vi "数据查询_数据查询.vi"() -> ()   [LabVIEW 2016]
uses:
  <vilib>/Utility/miscctls.llb/LVPointTypeDef.ctl
  <vilib>/Utility/miscctls.llb/LVRowAndColumnUnsignedTypeDef.ctl
  <userlib>/_OpenG.lib/array/array.llb/Sort 2D Array (String)__ogtk.vi
  <vilib>/addons/database/_DB Variant To Data/Database Variant To Data.xnode
panel:
  in  "导出":bool
  out "分钟小时":string(combo)="实时数据"
  out "工作类型":string(combo)="全部数据"
  in  "工作模式":string(combo)="全部数据"
  out "连接的字符串":string
  out "选中数据表":string
  in  "查询":bool
  in  "结束日期":string="2020/01/01"
  in  "起始日期":string="2010/01/01"
  out "XY图":cluster{"data":timestamp[], "data":dbl[]}[](graph)
  in  "组合框":string(combo)
  out "数据表":string[][](table)
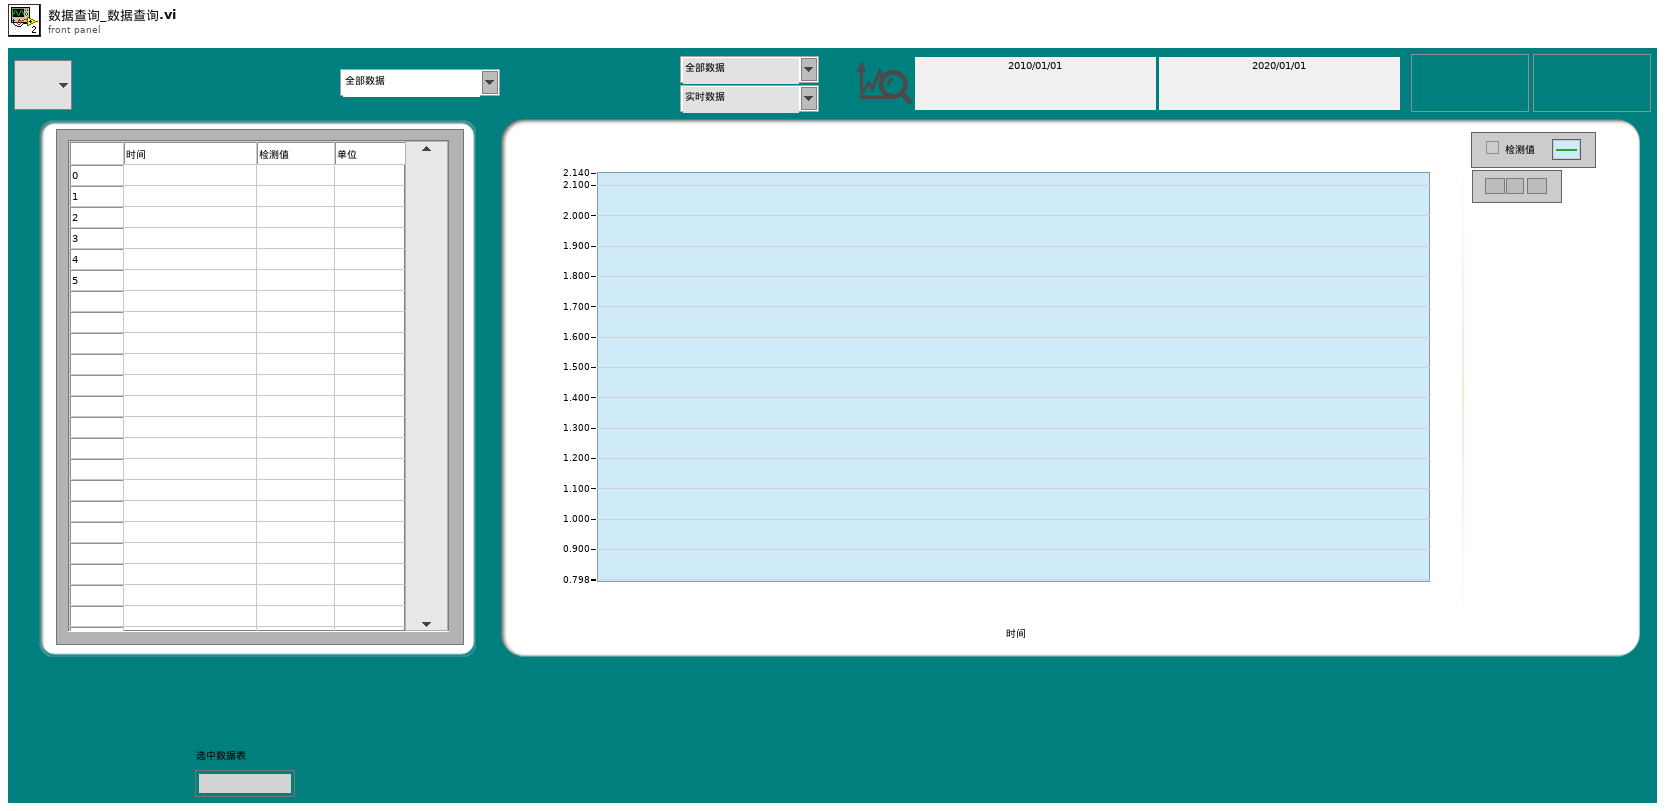
[diagram p1: front panel]
types:
  T1 = typedef "LVPointTypeDef.ctl" = cluster{"Horizontal":i16, "Vertical":i16}
  T2 = enum8{"Enabled", "Disabled", "Disabled and Grayed Out"}
  T3 = typedef "LVRowAndColumnUnsignedTypeDef.ctl" = cluster{"Row":u32, "Column":u32}
  T4 = typedef "LVPoint32TypeDef.ctl" = cluster{"Horizontal":i32, "Vertical":i32}
  T5 = typedef "LVPointDoubleTypeDef.ctl" = cluster{"Cursor X":dbl, "Cursor Y":dbl}
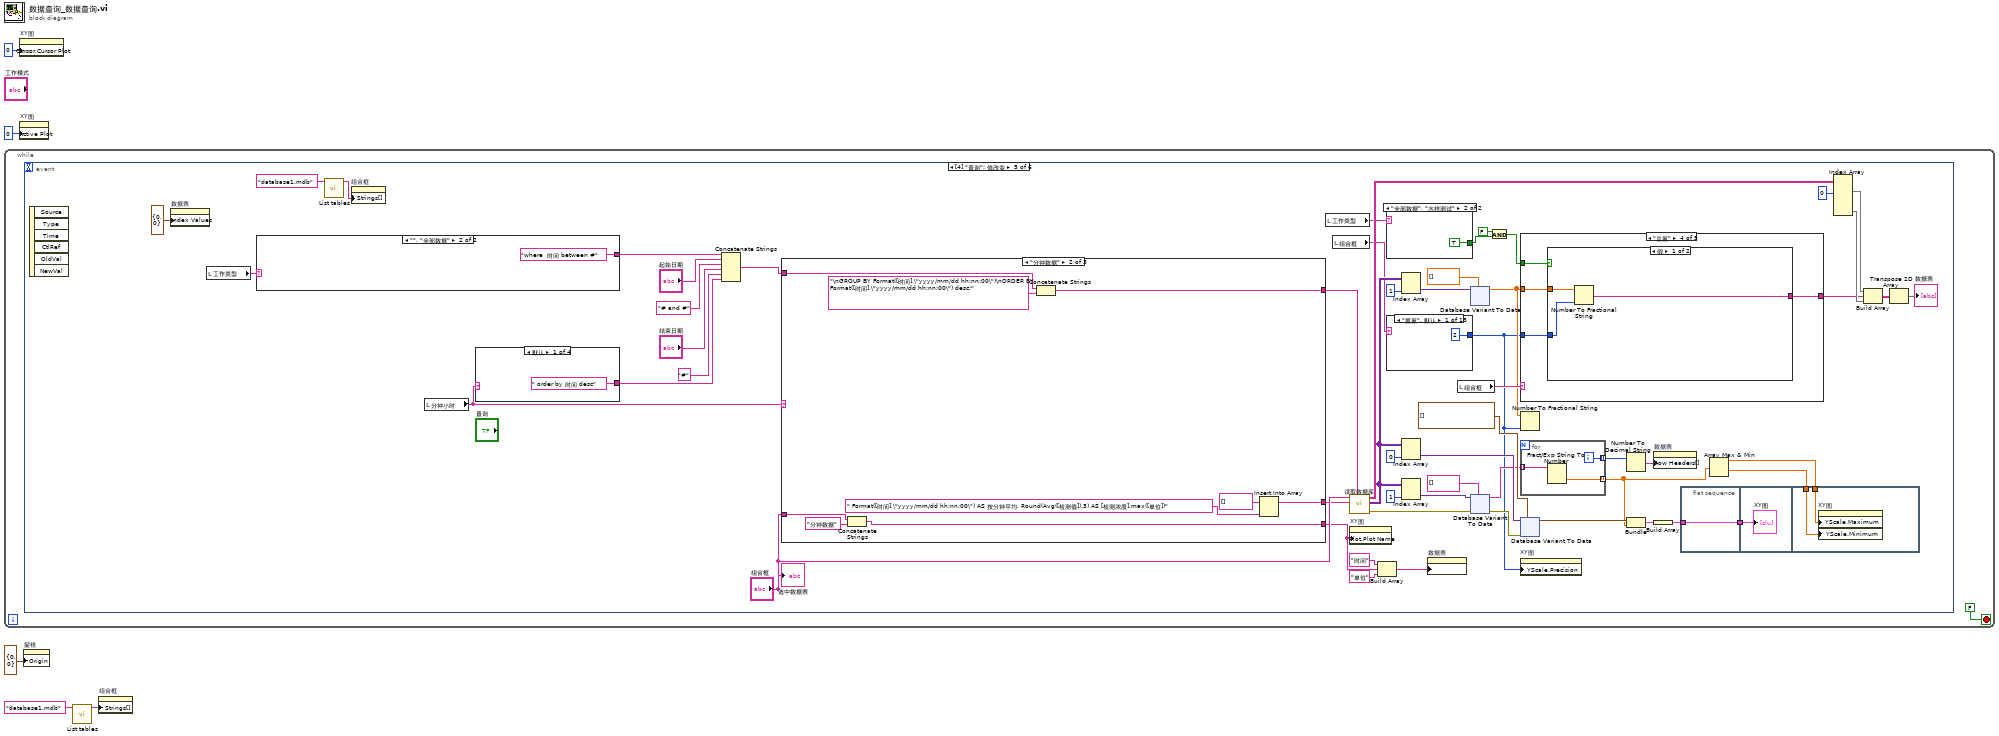
[diagram p0: block diagram]
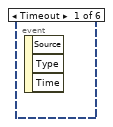
[diagram p2: hidden frame]
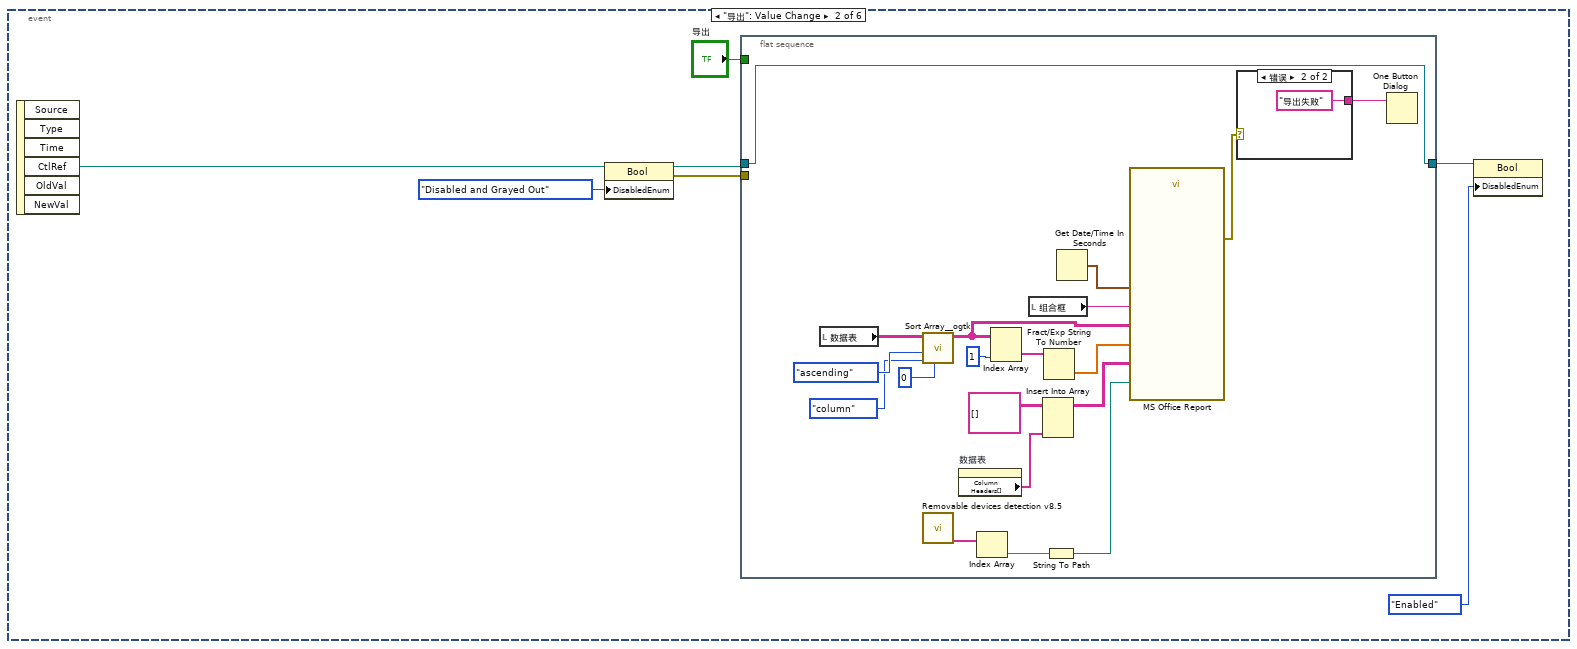
[diagram p3: hidden frame]
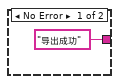
[diagram p4: hidden frame]
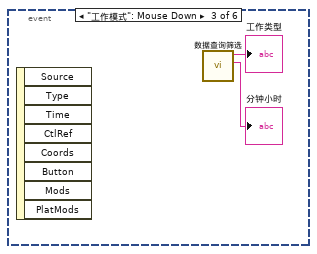
[diagram p5: hidden frame]
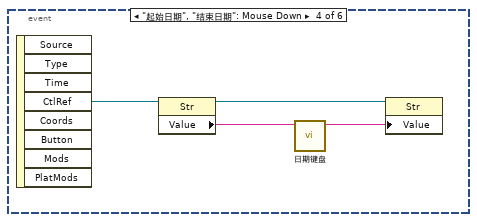
[diagram p6: hidden frame]
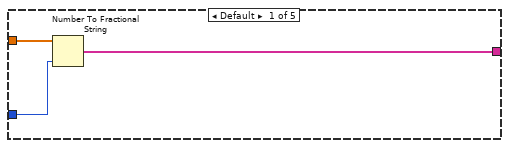
[diagram p8: hidden frame]
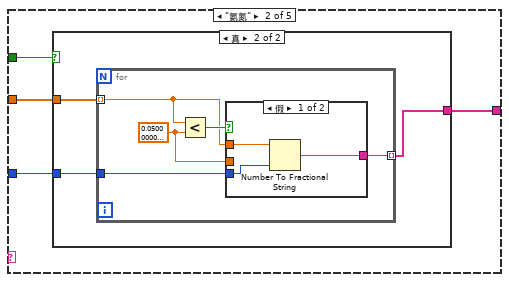
[diagram p9: hidden frame]
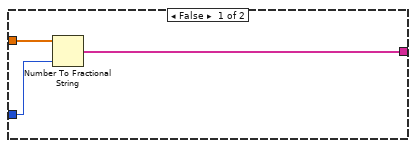
[diagram p10: hidden frame]
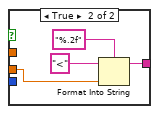
[diagram p11: hidden frame]
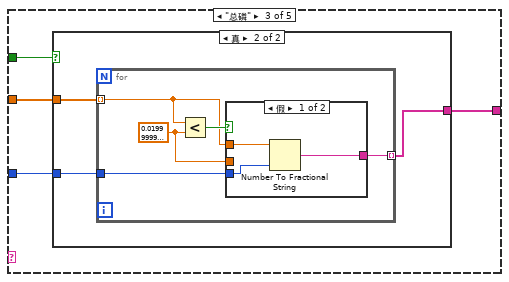
[diagram p12: hidden frame]
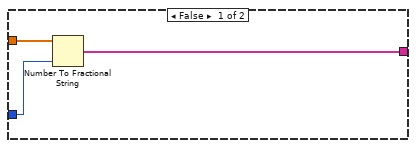
[diagram p13: hidden frame]
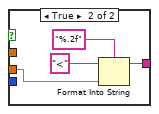
[diagram p14: hidden frame]
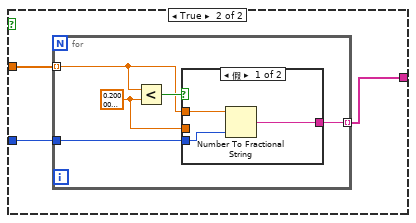
[diagram p15: hidden frame]
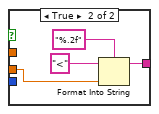
[diagram p16: hidden frame]
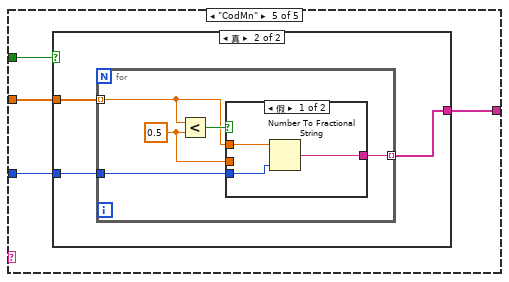
[diagram p17: hidden frame]
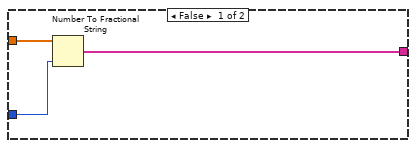
[diagram p18: hidden frame]
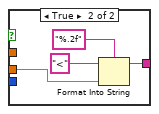
[diagram p19: hidden frame]
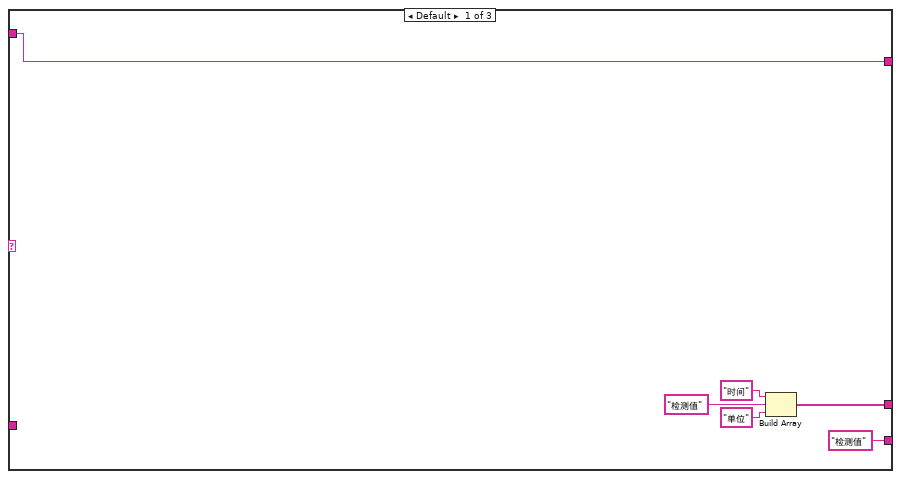
[diagram p20: hidden frame]
diagram:
  n1 = while {
    stop <- FALSE stop-if-true
    n2 = event shown="[4] \"查询\": 值改变" {
      selector: _ -> [_ _ _ _ _ _]
      dyn-events: _ -> [_ _ _ _ _ _]
      timeout: _ -> [_ _ _ _ _ _]
      event Timeout {
        n3 = event-data() -> ()  [unwired: 1 in, 3 out]
      }
      event "导出": Value Change {
        n4 = event-data() -> ("CtlRef"=w13:refnum<vi>)  [unwired: 1 in, 5 out]
        n5 = property class="Bool"(reference=w13, "DisabledEnum"=T2."Disabled and Grayed Out" ("禁用")) -> (reference out=w10:refnum<vi>, error out=w11:errorcluster)  [unwired: 1 in]
        n6 = flat-sequence {
          tunnel: w11 -> [_]
          tunnel: [w22] -> w9
          tunnel: w10 -> [w22]
          tunnel: "导出" -> [_]
          frame #0 {
            n7 = local read "数据表"() -> (w30:string[][])
            n8 = call-poly <userlib>:"Sort Array__ogtk.vi"("Column/Row to Sort By"=u32 0, "Sort By in"=enum16{"row", "column"}."column", "Order"=enum16{"ascending", "descending"}."ascending", "Array in"=w30) -> ("Sorted Array out"=w29:string[][])  [unwired: 4 in, 3 out]
            n9 = call "Removable devices detection v8.5.vi"() -> ("Removable"=w19:string[])  [unwired: 4 out]
            n10 = property on="数据表" class="Tbl (严格)"() -> ("Column Headers[]"=w15:string[])  [unwired: 2 in, 2 out]
            n11 = Index Array(array=w19) -> (element=w18:string)  [unwired: 1 in]
            n12 = Index Array(array=w29, index (col)=1 ("禁用的索引 (列)")) -> (element=w25:string[])  [unwired: 1 in]
            n13 = local read "组合框"() -> (w23:string)
            n14 = Insert Into Array(array=string[][] [], new element=w15) -> (w14:string[][])  [unwired: 2 in]
            n15 = Fract/Exp String To Number(string=w25) -> (number=w24:dbl[])  [unwired: 3 in, 1 out]
            n16 = String To Path(string=w18) -> (path=w17:path)
            n17 = Get Date/Time In Seconds() -> (seconds since 1Jan1904=w32:timestamp)
            n18 = call "MS Office Report"("Path to Save Report"=w17, "导出日期"=w32, "监测参数"=w23, "数据输入"=w29, "图表输入"=w24, "字段定义"=w14) -> ("error out"=w21:errorcluster)  [unwired: 20 in, 1 out]
            n19 = case shown="错误" w21 {
              tunnel: ["导出成功" ("消息") "导出失败" ("消息")] -> w20
              frame No Error {
              }
              frame Error {
              }
            }
            n20 = One Button Dialog(message=w20) -> ()  [unwired: 1 in, 1 out]
          }
        }
        n21 = property class="Bool"(reference=w9, "DisabledEnum"=T2."Enabled" ("禁用")) -> ()  [unwired: 1 in, 2 out]
      }
      event "工作模式": Mouse Down {
        n22 = event-data() -> ()  [unwired: 1 in, 8 out]
        n23 = call "数据查询筛选.vi"() -> ("分钟小时"=→"分钟小时":string, "工作类型"=→"工作类型":string)  [unwired: 10 in]
      }
      event "起始日期", "结束日期": Mouse Down {
        n24 = event-data() -> ("CtlRef"=w40:refnum<vi>)  [unwired: 1 in, 7 out]
        n25 = property class="Str"(reference=w40) -> (reference out=w38:refnum<vi>, "Value"=w39:string)  [unwired: 1 in, 1 out]
        n26 = call "日期键盘.vi"("原值"=w39) -> ("x+y"=w37:string)  [unwired: 10 in]
        n27 = property class="Str"(reference=w38, "Value"=w37) -> ()  [unwired: 1 in, 2 out]
      }
      event "查询": Value Change {
        n28 = event-data() -> ()  [unwired: 1 in, 6 out]
        n29 = property on="数据表" class="Tbl (严格)"("Index Values"=T3 {"Row"=0, "Column"=0} ("索引值")) -> ()  [unwired: 2 in, 2 out]
        n30 = local read "工作类型"() -> (w59:string)
        n31 = case shown="\"\", \"全部数据\"" w59 {
          selector: w59 -> [w216 _]
          tunnel: [w214 "where  时间 between #" ("condition")] -> w58
          frame Default {
            n32 = Format Into String(format string="where 测量模式 ='%s' and 时间 between #" ("condition"), w216) -> (resulting string=w214:string)  [unwired: 2 in, 1 out]
          }
          frame "", "全部数据" {
          }
        }
        n33 = call "List tables.vi"("database"="database1.mdb") -> ("tables"=w64:string[])  [unwired: 9 in, 1 out]
        n34 = property on="组合框" class="CmbBox"("Strings[]"=w64) -> ()  [unwired: 2 in, 2 out]
        n35 = local read "分钟小时"() -> (w55:string)
        n36 = case shown="默认" w55 {
          tunnel: [" order by 时间 desc" ("字符串") _ _ _] -> w57
          frame Default {
          }
          frame "分钟数据" {
          }
          frame "小时数据" {
          }
          frame "真" {
          }
        }
        n37 = Concatenate Strings(w58, "起始日期", "# and #" ("condition"), "结束日期", "#" ("condition"), w57) -> (w56:string)
        n38 = case shown="\"分钟数据\"" w55 {
          tunnel: [w190 w202 w207] -> w52
          tunnel: w56 -> [w194 w200 w209]
          tunnel: [w194 w199 w208] -> w54
          tunnel: ["检测值" w195 w204] -> w51
          tunnel: "组合框" -> [_ w196 w206]
          frame Default {
            n39 = Build Array("时间", "检测值", "单位" ("元素")) -> (w190:string[])
          }
          frame "分钟数据" {
            n40 = Concatenate Strings(w196, "分钟数据" ("字符串")) -> (w195:string)
            n41 = Concatenate Strings(w200, "\nGROUP BY Format([时间],\"yyyy/mm/dd hh:nn:00\")\nORDER BY Format([时间],\"yyyy/mm/dd hh:nn:00\") desc;" ("字符串")) -> (w199:string)
            n42 = Insert Into Array(array=string[] [] ("显示项"), new element=" Format([时间],\"yyyy/mm/dd hh:nn:00\") AS 按分钟平均, Round(Avg([检测值]),3) AS [检测浓度],max([单位])" ("新元素/子数组")) -> (w202:string[])  [unwired: 1 in]
          }
          frame "小时数据" {
            n43 = Concatenate Strings(w206, "小时数据" ("字符串")) -> (w204:string)
            n44 = Concatenate Strings(w209, "\nGROUP BY Format([时间],\"yyyy/mm/dd hh:00:00\")\nORDER BY Format([时间],\"yyyy/mm/dd hh:00:00\") desc;" ("字符串")) -> (w208:string)
            n45 = Insert Into Array(array=string[] [] ("显示项"), new element=" Format([时间],\"yyyy/mm/dd hh:00:00\") AS 按分钟平均, Round(Avg([检测值]),3) AS [检测浓度],max([单位])" ("新元素/子数组")) -> (w207:string[])  [unwired: 1 in]
          }
        }
        n46 = local read "工作类型"() -> (w44:string)
        n47 = local read "组合框"() -> (w65:string)
        n48 = call "读取数据库.vi"("condition"=w54, "显示项"=w52, "组合框"="组合框") -> ("error out"=w87:errorcluster, "data"=w70:variant[][], "表格"=w80:string[][])  [unwired: 5 in, 1 out]
        n49 = property on="XY图" class="XYGraph (严格)"("Plot.Plot Name"=w51) -> ()  [unwired: 2 in, 2 out]
        n50 = Build Array("时间", w51, "单位" ("元素")) -> (w74:string[])
        n51 = case shown="\"全部数据\", \"水样测试\"" w44 {
          tunnel: [_ TRUE] -> w43
          frame Default {
          }
          frame "全部数据", "水样测试" {
          }
        }
        n52 = case shown="\"氨氮\", 默认" w65 {
          tunnel: [i16 2 ("精度(6)") i16 1 ("精度(6)") i16 2 ("精度(6)") i16 2 ("精度(6)") i16 2 ("精度(6)") i16 2 ("精度(6)") i16 2 ("精度(6)") i16 2 ("精度(6)") i16 2 ("精度(6)") i16 2 ("精度(6)") i16 2 ("精度(6)") i16 1 ("精度(6)") i16 1 ("精度(6)")] -> w46
          frame "氨氮", Default {
          }
          frame "水温" {
          }
          frame "pH" {
          }
          frame "DO" {
          }
          frame "DOper" {
          }
          frame "电导率" {
          }
          frame "浊度" {
          }
          frame "藻密度" {
          }
          frame "叶绿素a" {
          }
          frame "总磷" {
          }
          frame "总氮" {
          }
          frame "CodCr" {
          }
          frame "CodMn" {
          }
        }
        n53 = Index Array(array=w70, index (col)=1 ("禁用的索引 (列)")) -> (element=w68:variant[])  [unwired: 1 in]
        n54 = Index Array(array=w70, index (col)=0 ("禁用的索引 (列)")) -> (element=w90:variant[])  [unwired: 1 in]
        n55 = Index Array(array=w70, index (col)=1 ("禁用的索引 (列)")) -> (element=w88:variant[])  [unwired: 1 in]
        n56 = property on="数据表" class="Tbl (严格)"("Column Headers[]"=w74) -> ()  [unwired: 2 in, 2 out]
        n57 = local read "组合框"() -> (w48:string)
        n58 = xnode "Database Variant To Data"("database variant"=w68, "type"=sgl[] []) -> ("data"=w47:sgl[])  [unwired: 1 in, 1 out]
        n59 = xnode "Database Variant To Data"("database variant"=w88, "error in (no error)"=w87, "type"=string[] []) -> ("data"=w73:string[], "error out"=w86:errorcluster)
        n60 = And(x=FALSE, y=w43) -> (x .and. y?=w42:bool)
        n61 = case shown="\"总氮\"" w48 {
          tunnel: w47 -> [w99 w104 w126 w147 w170]
          tunnel: w46 -> [w100 w102 w125 w148 w169]
          tunnel: [w98 w103 w124 w146 w168] -> w45
          tunnel: w42 -> [_ w101 w123 w145 w167]
          frame Default {
            n62 = Number To Fractional String(number=w99, precision (6)=w100) -> (F-format string=w98:string[])  [unwired: 2 in]
          }
          frame "氨氮" {
            n63 = case shown="真" w101 {
              tunnel: w104 -> [w107 w110]
              tunnel: [w105 w109] -> w103
              tunnel: w102 -> [w106 w108]
              frame False {
                n64 = Number To Fractional String(number=w107, precision (6)=w106) -> (F-format string=w105:string[])  [unwired: 2 in]
              }
              frame True {
                n65 = for {
                  tunnel: w110 -> [w112] mode=indexing
                  tunnel: [w113] -> w109 mode=indexing
                  tunnel: w108 -> [w111]
                  w114 = sgl 0.05 ("y")
                  n66 = Less?(x=w112, y=w114) -> (x < y?=w115:bool)
                  n67 = case shown="假" w115 {
                    tunnel: w114 -> [_ w121]
                    tunnel: [w116 w119] -> w113
                    tunnel: w112 -> [w118 _]
                    tunnel: w111 -> [w117 _]
                    frame False {
                      n68 = Number To Fractional String(number=w118, precision (6)=w117) -> (F-format string=w116:string)  [unwired: 2 in]
                    }
                    frame True {
                      n69 = Format Into String(format string="%.2f" ("格式字符串"), initial string="<" ("初始字符串"), w121) -> (resulting string=w119:string)  [unwired: 1 in, 1 out]
                    }
                  }
                }
              }
            }
          }
          frame "总磷" {
            n70 = case shown="真" w123 {
              tunnel: w126 -> [w129 w132]
              tunnel: w125 -> [w128 w131]
              tunnel: [w127 w130] -> w124
              frame False {
                n71 = Number To Fractional String(number=w129, precision (6)=w128) -> (F-format string=w127:string[])  [unwired: 2 in]
              }
              frame True {
                n72 = for {
                  tunnel: w132 -> [w134] mode=indexing
                  tunnel: [w135] -> w130 mode=indexing
                  tunnel: w131 -> [w133]
                  w136 = sgl 0.02 ("y")
                  n73 = Less?(x=w134, y=w136) -> (x < y?=w137:bool)
                  n74 = case shown="假" w137 {
                    tunnel: w136 -> [_ w143]
                    tunnel: [w138 w141] -> w135
                    tunnel: w134 -> [w140 _]
                    tunnel: w133 -> [w139 _]
                    frame False {
                      n75 = Number To Fractional String(number=w140, precision (6)=w139) -> (F-format string=w138:string)  [unwired: 2 in]
                    }
                    frame True {
                      n76 = Format Into String(format string="%.2f" ("格式字符串"), initial string="<" ("初始字符串"), w143) -> (resulting string=w141:string)  [unwired: 1 in, 1 out]
                    }
                  }
                }
              }
            }
          }
          frame "总氮" {
            n77 = case shown="假" w145 {
              tunnel: w148 -> [w151 w154]
              tunnel: w147 -> [w150 w153]
              tunnel: [w149 w152] -> w146
              frame False {
                n78 = Number To Fractional String(number=w150, precision (6)=w151) -> (F-format string=w149:string[])  [unwired: 2 in]
              }
              frame True {
                n79 = for {
                  tunnel: w153 -> [w156] mode=indexing
                  tunnel: [w157] -> w152 mode=indexing
                  tunnel: w154 -> [w155]
                  w158 = sgl 0.2 ("y")
                  n80 = Less?(x=w156, y=w158) -> (x < y?=w159:bool)
                  n81 = case shown="假" w159 {
                    tunnel: w158 -> [_ w165]
                    tunnel: [w160 w163] -> w157
                    tunnel: w156 -> [w162 _]
                    tunnel: w155 -> [w161 _]
                    frame False {
                      n82 = Number To Fractional String(number=w162, precision (6)=w161) -> (F-format string=w160:string)  [unwired: 2 in]
                    }
                    frame True {
                      n83 = Format Into String(format string="%.2f" ("格式字符串"), initial string="<" ("初始字符串"), w165) -> (resulting string=w163:string)  [unwired: 1 in, 1 out]
                    }
                  }
                }
              }
            }
          }
          frame "CodMn" {
            n84 = case shown="真" w167 {
              tunnel: w170 -> [w173 w176]
              tunnel: w169 -> [w172 w175]
              tunnel: [w171 w174] -> w168
              frame False {
                n85 = Number To Fractional String(number=w173, precision (6)=w172) -> (F-format string=w171:string[])  [unwired: 2 in]
              }
              frame True {
                n86 = for {
                  tunnel: w176 -> [w178] mode=indexing
                  tunnel: [w179] -> w174 mode=indexing
                  tunnel: w175 -> [w177]
                  w180 = sgl 0.5 ("y")
                  n87 = Less?(x=w178, y=w180) -> (x < y?=w181:bool)
                  n88 = case shown="假" w181 {
                    tunnel: w180 -> [_ w187]
                    tunnel: [w182 w185] -> w179
                    tunnel: w178 -> [w184 _]
                    tunnel: w177 -> [w183 _]
                    frame False {
                      n89 = Number To Fractional String(number=w184, precision (6)=w183) -> (F-format string=w182:string)  [unwired: 2 in]
                    }
                    frame True {
                      n90 = Format Into String(format string="%.2f" ("格式字符串"), initial string="<" ("初始字符串"), w187) -> (resulting string=w185:string)  [unwired: 1 in, 1 out]
                    }
                  }
                }
              }
            }
          }
        }
        n91 = Number To Fractional String(number=w47, precision (6)=w46) -> ()  [unwired: 2 in, 1 out]
        n92 = for {
          tunnel: w73 -> [w271] mode=indexing
          tunnel: [w270] -> w62 mode=indexing
          tunnel: [w269] -> w50 mode=indexing
          i -> [w269]
          n93 = Fract/Exp String To Number(string=w271) -> (number=w270:dbl)  [unwired: 3 in, 1 out]
        }
        n94 = xnode "Database Variant To Data"("database variant"=w90, "error in (no error)"=w86, "type"=timestamp[] []) -> ("data"=w81:timestamp[])  [unwired: 1 out]
        n95 = property on="XY图" class="XYGraph (严格)"("YScale.Precision"=w46) -> ()  [unwired: 2 in, 2 out]
        n96 = Number To Decimal String(number=w50) -> (decimal integer string=w49:string[])  [unwired: 1 in]
        n97 = Bundle("data"=w81, w62) -> (w82:cluster{"data":timestamp[], dbl[]})  [unwired: 1 in]
        n98 = property on="数据表" class="Tbl (严格)"("Row Headers[]"=w49) -> ()  [unwired: 2 in, 2 out]
        n99 = Build Array(w82) -> (w83:cluster{"data":timestamp[], dbl[]}[])
        n100 = flat-sequence {
          tunnel: [w272] -> w84
          tunnel: w83 -> [w272]
          tunnel: w84 -> [w273]
          tunnel: w61 -> [w275]
          tunnel: w60 -> [w274]
          frame #0 {
          }
          frame #1 {
            "XY图" <- w273
          }
          frame #2 {
            n101 = property on="XY图" class="XYGraph (严格)"("YScale.Maximum"=w275, "YScale.Minimum"=w274) -> ()  [unwired: 2 in, 2 out]
          }
        }
        n102 = Array Max & Min(array=w62) -> (max value=w61:dbl, min value=w60:dbl)  [unwired: 2 out]
        n103 = Index Array(array=w80, index (col) #1=0 ("禁用的索引 (列)")) -> (element #1=w78:string[], element #3=w71:string[])  [unwired: 5 in, 1 out]
        n104 = Build Array(w78, w45, w71) -> (w77:string[][])
        n105 = Transpose 2D Array(2D array=w77) -> (transposed array=→"数据表":string[][])
        "选中数据表" <- "组合框"
      }
      event "XY图": Mouse Move {
        w370 = "   " ("字符串")
        n106 = event-data() -> ("CtlRef"=w380:refnum<vi>, "Coords"=w379:T4)  [unwired: 1 in, 3 out]
        n107 = invoke class="XYGraph (严格)" method="Map Coords To XY"(reference=w380, "Coords"=w379) -> (reference out=w378:refnum<vi>, error out=w375:errorcluster, "XY"=w377:cluster{"X":dbl, "Y":dbl})  [unwired: 5 in, 4 out]
        n108 = property class="XYGraph (严格)"(reference=w378, error in=w375, "Cursor.Cursor Position"=w377) -> (error out=w376:errorcluster)  [unwired: 1 out]
        n109 = property on="XY图" class="XYGraph (严格)"(error in=w376) -> ("Cursor.Cursor Position"=w373:T5, "YScale.Precision"=w366:u8)  [unwired: 1 in, 2 out]
        n110 = Unbundle(w373) -> ("Cursor X"=w372:dbl, "Cursor Y"=w369:dbl)
        n111 = property on="XY图" class="XYGraph (严格)"() -> ("Plot.Plot Name"=w367:string)  [unwired: 2 in, 2 out]
        n112 = Number To Fractional String(number=w369, precision (6)=w366) -> (F-format string=w368:string)  [unwired: 2 in]
        n113 = Format Date/Time String(seconds (now)=w372) -> (date/time string=w371:string)  [unwired: 2 in]
        n114 = Concatenate Strings(w367, w370, w371, w370, w368) -> (→"连接的字符串":string)
      }
    }
  }
  n115 = property on="XY图" class="XYGraph (严格)"("Cursor.Cursor Plot"=0 ("游标.游标关联曲线")) -> ()  [unwired: 2 in, 2 out]
  n116 = property on="XY图" class="XYGraph (严格)"("Active Plot"=u32 0 ("活动曲线")) -> ()  [unwired: 2 in, 2 out]
  n117 = property on="窗格" class="Pane"("Origin"=T1 {"Horizontal"=0, "Vertical"=0} ("原点")) -> ()  [unwired: 2 in, 2 out]
  n118 = call "List tables.vi"("database"="database1.mdb") -> ("tables"=w1:string[])  [unwired: 9 in, 1 out]
  n119 = property on="组合框" class="CmbBox"("Strings[]"=w1) -> ()  [unwired: 2 in, 2 out]
